vi "Read OPC UA Client Refnum.vi"(8 "error in (no error)":errorcluster, 11 "UA Server in":refnum<class "UA Server.lvclass">) -> (0 "error out":errorcluster, 2 "Server Connection Information.Server Endpoint URL":string, 3 "UA Server out":refnum<class "UA Server.lvclass">)   [LabVIEW 2017, in "opcua.lvlib" / "Browser Core.lvlib" / "UA Server.lvclass"]
uses:
  UA Server.lvclass
  UA Server.lvclass/UA Server.ctl
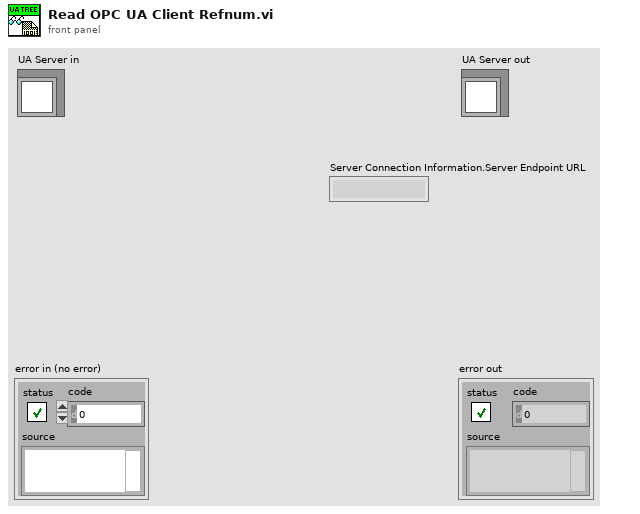
[diagram p1: front panel]
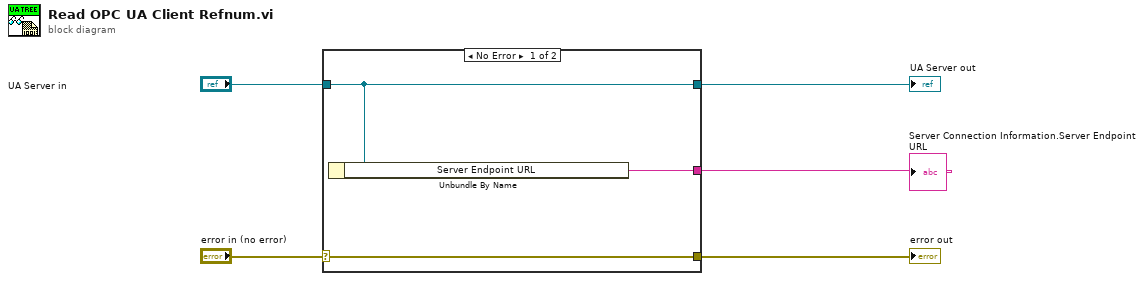
[diagram p0: block diagram]
diagram:
  n1 = case shown="No Error" "error in (no error)" {
    selector: "error in (no error)" -> [w8 w9]
    tunnel: [w8 w9] -> w4
    tunnel: [w7 w10] -> w2
    tunnel: "UA Server in" -> [w7 w10]
    tunnel: [w6 _] -> w1
    frame No Error {
      n2 = Unbundle By Name(w7) -> ("Server Endpoint URL"=w6:string)
    }
    frame Error {
    }
  }
  "error out" <- w4
  "UA Server out" <- w2
  "Server Connection Information.Server Endpoint URL" <- w1
